vi "Actor Core.vi"(8 "error in":errorcluster, 11 "Generator in":refnum<class "Generator.lvclass">) -> (0 "error out":errorcluster, 3 "Actor out":refnum<class "Actor.lvclass">)   [LabVIEW 2018, in "Generator Actor.lvlib" / "Generator.lvclass"]
doc: "(<B>Filename</B>: Actor Framework.lvlib:Actor.lvclass:Actor Core.vi)\n\nReceives messages to the actor, reacts to them, and initiates any error handling that may shut the actor down.\n\nDescendant classes may override this VI to append parallel tasks for the actor to complete while it handles messages. Overrides use the Call Parent Method node."
uses:
  Generator.lvclass
  C:/Users/Administrator/Desktop/2018LabVIEW EMS/EMS Generic Actor/EMS Generic/EMS Generic.lvclass
  <vilib>/ActorFramework/Actor/Actor.lvclass
  EMS Generic Actor/EMS Generic/EMS Generic.lvclass/EMS Generic.ctl
  <vilib>/ORNL/CSEISMIC DDS/CSEISMIC DDS Base/CSEISMIC DDS.lvclass/CSEISMIC DDS.ctl
  <vilib>/ORNL/CSEISMIC DDS/CSEISMIC DDS Base/Accessors/Write DDS Reference.vi
  <vilib>/ORNL/CSEISMIC DDS/CSEISMIC DDS Base/Accessors/Read DDS Reference.vi
  <vilib>/ORNL/CSEISMIC DDS/DDS Reader/DDS Reader.lvclass
  C:/Program Files (x86)/National Instruments/LabVIEW 2018/vi.lib/ORNL/CSEISMIC DDS/CSEISMIC DDS Base/CSEISMIC DDS.lvclass
  <vilib>/ORNL/CSEISMIC DDS/CSEISMIC DDS Base/Error Handler.vi
  Device DDS Communications Framework/Device DDS Communications/Device DDS Communications.lvclass
  EMS Generic Actor/EMS Generic/EMS Generic.lvclass
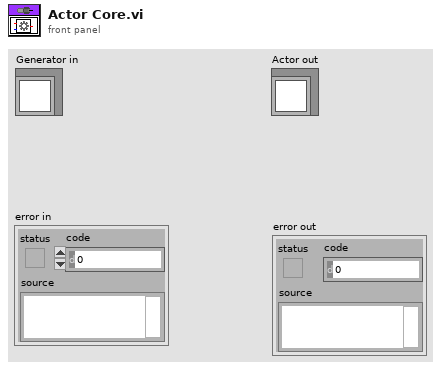
[diagram p1: front panel]
types:
  T1 = typedef "CSEISMIC DDS.lvlib/CSEISMIC DDS.lvclass/DeviceID.ctl" = string
  T2 = typedef "CSEISMIC DDS.lvlib/CSEISMIC DDS.lvclass/Generator_Info.ctl" = cluster{"DeviceID":T1, "Voltage (V)":dbl, "MinimumPower (kVA)":dbl, "EnergyRating (kWh)":dbl, "RampRate (kW/s)":dbl, "MaxPowerFactorLeading":dbl, "MaxPowerFactorLagging":dbl, "EfficiencyCurve":T3, "StartCost":dbl, "FuelCost":dbl, "StartTime (s)":dbl}
  T3 = typedef "CSEISMIC DDS.lvlib/CSEISMIC DDS.lvclass/EfficiencyCurve.ctl" = cluster{"Power (kW)":dbl[], "Efficiency (%)":dbl[]}
  T4 = typedef "LVDDS_library.lvlib/DDS Sample Info.ctl" = cluster{"DDS_SampleStateKind":enum32{"DDS_INVALID_SAMPLE_STATE", "DDS_READ_SAMPLE_STATE", "DDS_NOT_READ_SAMPLE_STATE"}, "DDS_ViewStateKind":enum32{"DDS_INVALID_SAMPLE_STATE", "DDS_NEW_VIEW_STATE", "DDS_NOT_NEW_VIEW_STATE"}, "DDS_InstanceStateKind":enum32{"DDS_INVALID_STATE", "DDS_ALIVE_INSTANCE_STATE", "DDS_NOT_ALIVE_DISPOSED_INSTANCE_STATE", "", "DDS_NOT_ALIVE_NO_WRITERS_INSTANCE_STATE"}, "sec":i32, "nanosec":u32, "valid_data":bool}
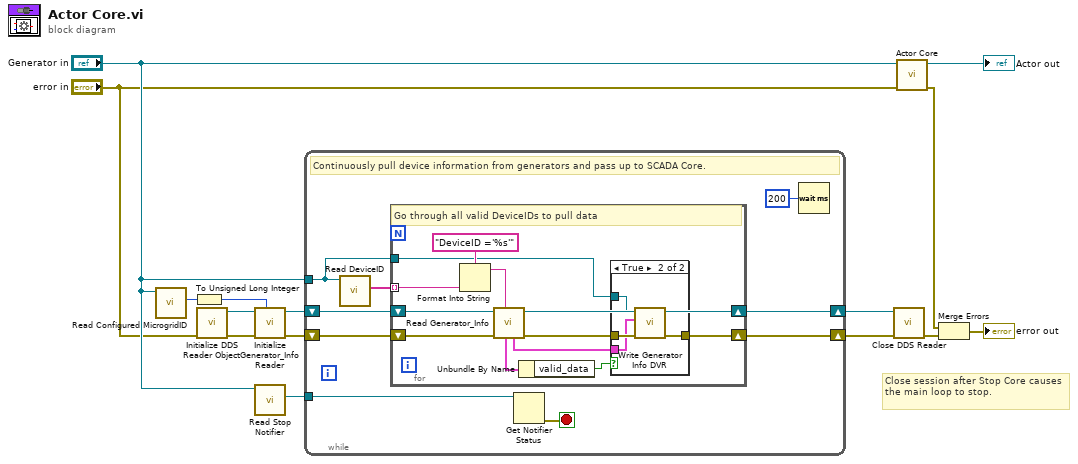
[diagram p0: block diagram]
diagram:
  # "Close session after Stop Core causes the main loop to stop."
  n1 = call "Read Configured MicrogridID.vi"("EMS Generic in"="Generator in") -> ("Microgrid ID"=w14:u8)  [unwired: 8 in, 2 out]
  n2 = To Unsigned Long Integer(number=w14) -> (unsigned 32bit integer=w2:u32)
  n3 = call <vilib>:"Initialize DDS Reader Object.vi"("error in"="error in") -> ("error out"=w11:errorcluster, "DDS Reader out"=w10:refnum<class "DDS Reader.lvclass">)  [unwired: 9 in]
  n4 = call <vilib>:"Initialize Generator_Info Reader.vi"("MicrogridID"=w2, "error in"=w11, "DDS Reader in"=w10) -> ("error out"=w9:errorcluster, "DDS Reader out"=w8:refnum<class "DDS Reader.lvclass">)  [unwired: 7 in]
  n5 = call "Read Stop Notifier.vi"("EMS Generic in"="Generator in") -> ("stop"=w4:refnum<notifier>)  [unwired: 9 in, 1 out]
  n6 = while {
    tunnel: w4 -> [w24]
    shift-right: [w18] -> w6
    shift-left: w9 -> [w20]
    shift-right: [w17] -> w7
    shift-left: w8 -> [w19]
    tunnel: "Generator in" -> [w16]
    stop <- w23 stop-if-true
    # "Continuously pull device information from generators and pass up to SCADA Core."
    n7 = call-dynamic "Read DeviceID.vi"("Device DDS Communications in"=w16) -> ("DeviceID"=w21:T1[])  [unwired: 9 in, 1 out]
    n8 = for {
      shift-right: [w35] -> w17
      shift-left: w19 -> [w36]
      shift-right: [w26] -> w18
      shift-left: w20 -> [w34]
      tunnel: w21 -> [w32] mode=indexing
      tunnel: w16 -> [w25]
      # "Go through all valid DeviceIDs to pull data"
      n9 = Format Into String(format string="DeviceID ='%s'", w32) -> (resulting string=w31:string)  [unwired: 2 in, 1 out]
      n10 = call <vilib>:"Read Generator_Info.vi"("Query condition"=w31, "error in"=w34, "DDS Reader in"=w36) -> ("error out"=w27:errorcluster, "DDS Reader out"=w35:refnum<class "DDS Reader.lvclass">, "data"=w28:T2, "DDS Sample Info"=w30:T4)  [unwired: 5 in]
      n11 = Unbundle By Name(w30) -> ("valid_data"=w29:bool)
      n12 = case shown="True" w29 {
        tunnel: w28 -> [_ w39]
        tunnel: w27 -> [w37 w41]
        tunnel: [w37 w40] -> w26
        tunnel: w25 -> [_ w38]
        frame False {
        }
        frame True {
          n13 = call "Write Generator Info DVR.vi"("error in"=w41, "Generator_Info"=w39, "EMS Generic in"=w38) -> ("error out"=w40:errorcluster)  [unwired: 7 in, 1 out]
        }
      }
    }
    n14 = Get Notifier Status(notifier=w24) -> (error out=w23:errorcluster)  [unwired: 1 in, 4 out]
    n15 = Wait (ms)(milliseconds to wait=u32 200) -> ()  [unwired: 1 out]
  }
  n16 = call <vilib>:"Close DDS Reader.vi"("error in"=w6, "DDS Reader in"=w7) -> ("error out"=w5:errorcluster)  [unwired: 9 in]
  n17 = call-parent "Actor Core.vi"("error in"="error in", "Actor in"="Generator in") -> ("error out"=w15:errorcluster, "Actor out"=→"Actor out":refnum<class "Actor.lvclass">)  [unwired: 8 in]
  n18 = Merge Errors(w15, w5) -> (→"error out":errorcluster)
